vi "New - DragStart.vi"(8 "error in (no error)":errorcluster, 10 "DragStart Indices":i32[](array[numeric]), 11 "Ref":refnum<vi>) -> (0 "error out":errorcluster, 3 "BetterDropOp out":refnum<class "BetterDropOp.lvclass">)   [LabVIEW 2020, in "BetterDragAndDrop.lvlib" / "BetterDropOp.lvclass"]
uses:
  BetterDropOp.lvclass
  BetterDropOp.lvclass/BetterDropOp.ctl
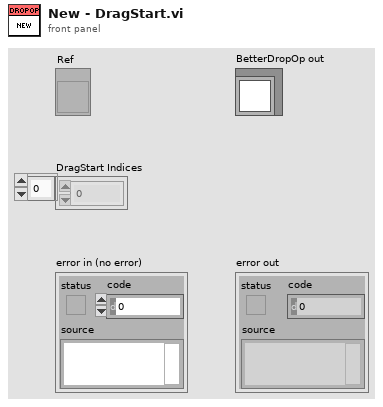
[diagram p1: front panel]
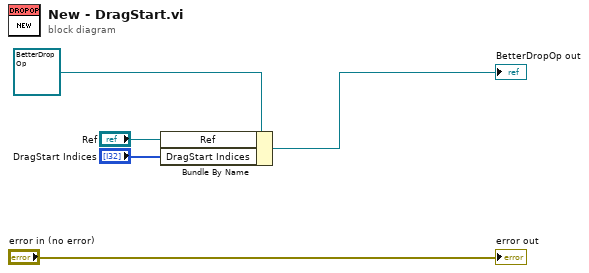
[diagram p0: block diagram]
diagram:
  n1 = Bundle By Name(cluster=refnum<class "BetterDropOp.lvclass"> refnum ("BetterDragStart out"), "Ref"="Ref", "DragStart Indices"="DragStart Indices") -> (→"BetterDropOp out":refnum<class "BetterDropOp.lvclass">)
  "error out" <- "error in (no error)"
